vi "Configure Runt Trigger Source [RT].vi"(0 "CS++Scope":refnum<class "CS++Scope.lvclass">, 5 "trigger source (\"CHANNEL1\")":string(combo)="CHANNEL1", 7 "runt low threshold (1.0 V)":dbl[unit]=1.0 format="%.3f", 9 "runt high threshold (4.0 V)":dbl[unit]=4.0 format="%.3f", 11 "error in (no error)":errorcluster) -> (4 "CS++Scope out":refnum<class "CS++Scope.lvclass">, 15 "error out":errorcluster)   [LabVIEW 2013, in "CS++Scope.lvlib" / "CS++Scope.lvclass"]
doc: "This VI configures the runt trigger. A runt trigger occurs when the trigger signal you specify with the Runt Trigger Source parameter crosses one of the runt thresholds twice without crossing the other runt threshold. You specify the runt thresholds with the Runt Low Threshold and Runt High Threshold parameters. You specify the polarity of the runt with the Runt Polarity parameter.\n\nNote \n(1) This VI affects instrument behavior only if the trigger type is\n IVISCOPE_VAL_RUNT_TRIGGER. Call the IviScope Configure Trigger\n and IviScope Configure Trigger Coupling VIs to set the trigger type and\n trigger coupling before calling this VI.\n\n(2) This VI is part of the IviScopeRuntTrigger [RT] extension group."
uses:
  CS++Scope.lvclass
  CSPP_Core/Classes/CS++ProcessVariables/ProcessVariable/PV.lvclass
  PV-Enum.ctl
  CS++Scope.lvclass/CS++Scope.ctl
  CSPP_Core/Classes/CS++ProcessVariables/PVConnection/PVConnection.lvclass
  CSPP_Core/Classes/CS++ProcessVariables/ProcessVariable/PV.lvclass/PV.ctl
  CSPP_Core/Classes/CS++ProcessVariables/ProcessVariable/Write Data.vi
  CSPP_Core/Classes/CS++ProcessVariables/ProcessVariable/Write Timestamp.vi
  CSPP_Core/Classes/CS++ProcessVariables/ProcessVariable/Write Quality.vi
  CSPP_Core/Classes/CS++ProcessVariables/ProcessVariable/Write status.vi
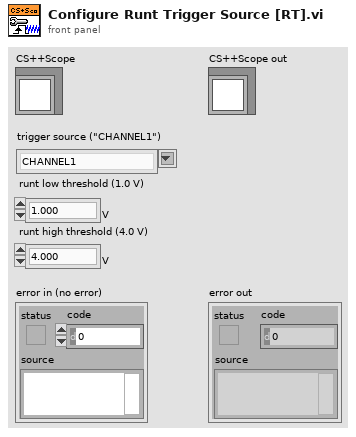
[diagram p1: front panel]
types:
  T1 = typedef "CS++Scope.lvlib/CS++Scope.lvclass/PV-Enum.ctl" = enum16{"ActualSampleRate", "TimePerRecord", "AcquisitionStartTime", "TriggerLevel", "GlitchWidth", "LowReference", "MidReference", "HighReference", "RuntLowThreshold", "RuntHighThreshold", "TriggerHoldoff", "WidthLowThreshold", "WidthHighThreshold", "AcquisitionStatus", "ActualRecordLength", "ActualSampleMode", "ACLineTriggerSlope", "MinRecordLength", "AcquisitionType", "TriggerSlope", "GlitchCondition", "GlitchPolarity", "InterpolationMethod", "NumberOfAverages", "NumberOfEnvelopes", "TriggerType", "TriggerCoupling", "TriggerModifier", "TVLineNumber", "TVEvent", "TVTriggerPolarity", "TVSignalFormat", "WidthCondition", "WidthPolarity", "MeasurementDone", "ContinousAcquisition", "TriggerSource", "Waveform"}
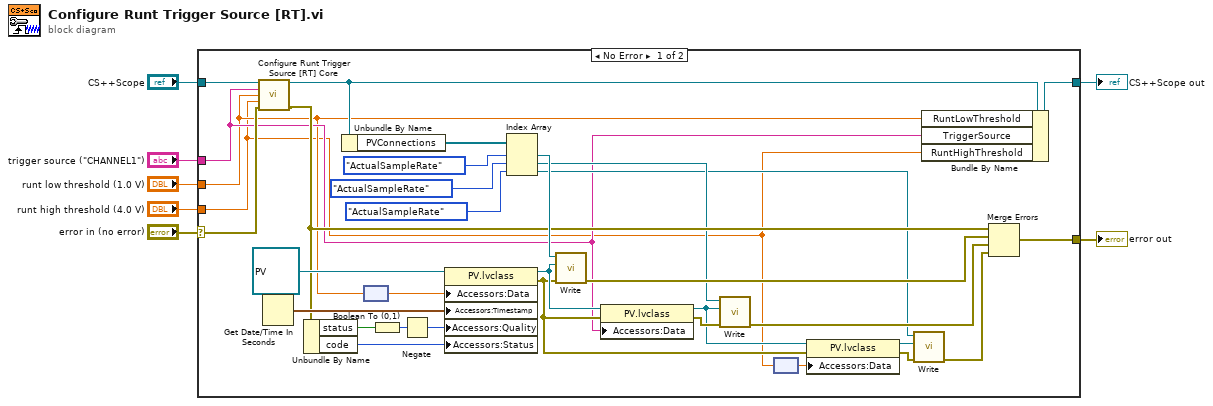
[diagram p0: block diagram]
diagram:
  n1 = case shown="No Error" "error in (no error)" {
    selector: "error in (no error)" -> [w14 w42]
    tunnel: [w13 w42] -> w6
    tunnel: [w15 w41] -> w2
    tunnel: "CS++Scope" -> [w16 w41]
    tunnel: "trigger source (\"CHANNEL1\")" -> [w12 _]
    tunnel: "runt low threshold (1.0 V)" -> [w11 _]
    tunnel: "runt high threshold (4.0 V)" -> [w9 _]
    frame No Error {
      n2 = call-dynamic "Configure Runt Trigger Source [RT] Core.vi"("CS++Scope"=w16, "trigger source (\"CHANNEL1\")"=w12, "runt low threshold (1.0 V)"=w11, "runt high threshold (4.0 V)"=w9, "error in (no error)"=w14) -> ("CS++Scope out"=w30:refnum<class "CS++Scope.lvclass">, "error out"=w29:errorcluster)  [unwired: 9 in]
      n3 = Get Date/Time In Seconds() -> (seconds since 1Jan1904=w35:timestamp)
      n4 = Unbundle By Name(w29) -> ("status"=w38:bool, "code"=w39:i32)
      n5 = Unbundle By Name(w30) -> ("PVConnections"=w34:refnum<class "PVConnection.lvclass">[])
      n6 = node(w11) -> (w10:dbl)
      n7 = Boolean To (0,1)(Boolean=w38) -> (0, 1=w37:i16)
      n8 = Negate(x=w37) -> (-x=w36:i16)
      n9 = property class="PV.lvclass"(reference=refnum<class "PV.lvclass"> refnum ("CS++ProcessVariables.lvlib:PV.lvclass"), "Accessors:Data"=w10, "Accessors:Timestamp"=w35, "Accessors:Quality"=w36, "Accessors:Status"=w39) -> (reference out=w24:refnum<class "PV.lvclass">, error out=w20:errorcluster)  [unwired: 1 in]
      n10 = Index Array(array=w34, index #1=PV-Enum."ActualSampleRate" ("PV-Enum"), index #2=PV-Enum."ActualSampleRate" ("PV-Enum"), index #3=PV-Enum."ActualSampleRate" ("PV-Enum")) -> (element #1=w32:refnum<class "PVConnection.lvclass">, element #2=w22:refnum<class "PVConnection.lvclass">, element #3=w18:refnum<class "PVConnection.lvclass">)
      n11 = call-dynamic "Write.vi"("error in (no error)"=w20, "PV"=w24, "PVConnection in"=w32) -> ("error out"=w31:errorcluster)  [unwired: 7 in, 1 out]
      n12 = property class="PV.lvclass"(reference=w24, error in=w20, "Accessors:Data"=w12) -> (reference out=w21:refnum<class "PV.lvclass">, error out=w23:errorcluster)
      n13 = call-dynamic "Write.vi"("error in (no error)"=w23, "PV"=w21, "PVConnection in"=w22) -> ("error out"=w26:errorcluster)  [unwired: 7 in, 1 out]
      n14 = node(w9) -> (w8:dbl)
      n15 = property class="PV.lvclass"(reference=w21, error in=w20, "Accessors:Data"=w8) -> (reference out=w19:refnum<class "PV.lvclass">, error out=w17:errorcluster)
      n16 = call-dynamic "Write.vi"("error in (no error)"=w17, "PV"=w19, "PVConnection in"=w18) -> ("error out"=w25:errorcluster)  [unwired: 7 in, 1 out]
      n17 = Bundle By Name(cluster=w30, "RuntLowThreshold"=w11, "TriggerSource"=w12, "RuntHighThreshold"=w9) -> (w15:refnum<class "CS++Scope.lvclass">)
      n18 = Merge Errors(w29, w31, w26, w25) -> (w13:errorcluster)
    }
    frame Error {
    }
  }
  "error out" <- w6
  "CS++Scope out" <- w2
